vi "frequency_phase_plot.vi"() -> ()   [LabVIEW 2014]
uses:
  <vilib>/Analysis/baseanly.llb/Mean (DBL).vi
  <userlib>/Nanonis Prog Interface V5/Nanonis Prog Interface.lvlib
  <vilib>/Analysis/NI_AALBase.lvlib
panel:
  out "XY Graph":cluster{"X":dbl[], "Y":dbl[]}[](graph)
  out "Array":cluster{dbl, dbl}[](array[cluster])
  out "phase":dbl[](array[numeric])
  out "freq":dbl[](array[numeric])
  out "Step Size":dbl
  in  "Integration Time (ms)":i32
  in  "Settling Time (ms)":i32
  in  "Number of Points":i32
  in  "End Frequency (Hz)":sgl
  in  "Start Frequency (Hz)":sgl
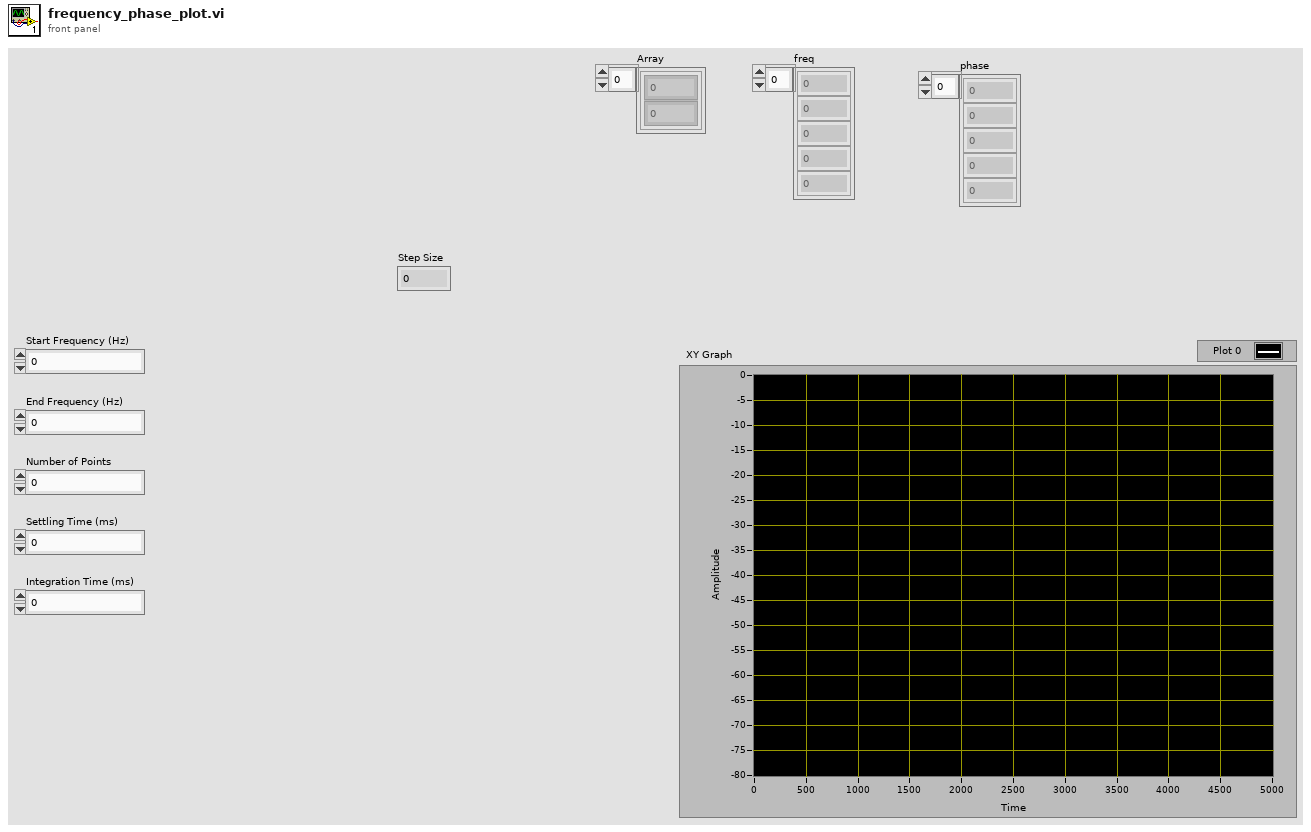
[diagram p1: front panel]
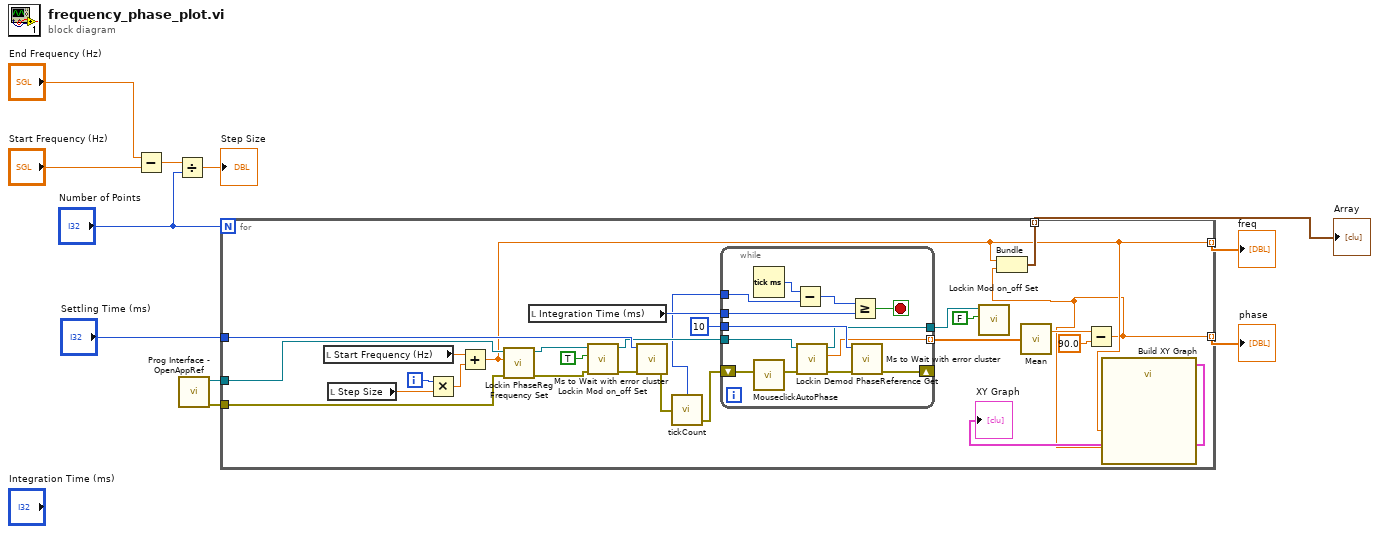
[diagram p0: block diagram]
diagram:
  n1 = Subtract(x="End Frequency (Hz)", y="Start Frequency (Hz)") -> (x-y=w8:sgl)
  n2 = Divide(x=w8, y="Number of Points") -> (x/y=→"Step Size":sgl)
  n3 = call <userlib>:"Prog Interface - OpenAppRef.vi"() -> ("Error out"=w5:errorcluster, "Application reference"=w6:refnum<vi>)  [unwired: 6 in]
  n4 = for {
    N: "Number of Points" -> [_]
    tunnel: w6 -> [w34]
    tunnel: w5 -> [w33]
    tunnel: "Settling Time (ms)" -> [w24]
    tunnel: [w12] -> w2 mode=indexing
    tunnel: [w13] -> w3 mode=indexing
    tunnel: [w18] -> w1 mode=indexing
    i -> [w29]
    n5 = local read "Start Frequency (Hz)"() -> (w37:sgl)
    n6 = local read "Step Size"() -> (w36:dbl)
    n7 = Multiply(x=w29, y=w36) -> (x*y=w35:dbl)
    n8 = Add(x=w37, y=w35) -> (x+y=w13:dbl)
    n9 = call <userlib>:"Lockin PhaseReg Frequency Set.vi"("Error in (no error)"=w33, "Frequency (Hz)"=w13, "Application ref in"=w34) -> ("Error out"=w32:errorcluster, "Application ref out"=w31:refnum<vi>)  [unwired: 7 in]
    n10 = local read "Integration Time (ms)"() -> (w20:i32)
    n11 = call <userlib>:"Lockin Mod on_off Set.vi"("Error in (no error)"=w32, "Lockin ON/OFF"=TRUE, "Application ref in"=w31) -> ("Error out"=w25:errorcluster, "Application ref out"=w23:refnum<vi>)  [unwired: 7 in]
    n12 = call <userlib>:"Ms to Wait with error cluster.vi"("error in (no error)"=w25, "milliseconds to wait"=w24) -> ("error out"=w17:errorcluster)  [unwired: 4 in, 1 out]
    n13 = call "tickCount.vi"("error in (no error)"=w17) -> ("error out"=w16:errorcluster, "millisecond timer value"=w15:u32)
    n14 = while {
      tunnel: w23 -> [w40]
      tunnel: [w38] -> w22 mode=indexing
      tunnel: w15 -> [w50]
      tunnel: 10 ("Integration Time (ms)") -> [w46]
      tunnel: w20 -> [w45]
      shift-right: [w44] -> _
      shift-left: w16 -> [w43]
      tunnel: [w39] -> w19
      stop <- w47 stop-if-true
      n15 = Tick Count (ms)() -> (millisecond timer value=w49:u32)
      n16 = call "MouseclickAutoPhase.vi"("error in (no error)"=w43) -> ("error out"=w42:errorcluster)  [unwired: 10 in]
      n17 = Subtract(x=w49, y=w50) -> (x-y=w48:u32)
      n18 = call <userlib>:"Lockin Demod PhaseReference Get.vi"("Error in (no error)"=w42, "Application ref in"=w40) -> ("Error out"=w41:errorcluster, "Phase Reference"=w38:sgl, "Application ref out"=w39:refnum<vi>)  [unwired: 7 in]
      n19 = Greater Or Equal?(x=w48, y=w45) -> (x >= y?=w47:bool)
      n20 = call <userlib>:"Ms to Wait with error cluster.vi"("error in (no error)"=w41, "milliseconds to wait"=w46) -> ("error out"=w44:errorcluster)  [unwired: 4 in, 1 out]
    }
    n21 = call <userlib>:"Lockin Mod on_off Set.vi"("Lockin ON/OFF"=FALSE, "Application ref in"=w19) -> ()  [unwired: 8 in, 2 out]
    n22 = call-poly <vilib>:"Mean.vi"("X"=w22) -> ("mean"=w27:dbl)  [unwired: 1 out]
    n23 = Subtract(x=w27, y=90.0) -> (x-y=w12:dbl)
    n24 = Bundle(w13, w12) -> (w18:cluster{dbl, dbl})  [unwired: 1 in]
    n25 = call "Build XY Graph"("Y Input"=w12, "X Input"=w13) -> ("XY Graph"=→"XY Graph":cluster{"X":dbl[], "Y":dbl[]}[])  [unwired: 8 in, 1 out]
  }
  "freq" <- w3
  "phase" <- w2
  "Array" <- w1
